vi "Testing.vi"() -> ()   [LabVIEW 2019]
panel:
  in  "process parameters":T1={"static gain"=2.5, "lag (s)"=2.5, "deadtime (s)"=0.001, "load"=0.0, "deadband"=0.0, "sensor noise"=0.0, "initial PV"=30.0, "plant noise"=0.0} {"plant noise" format="%.2f"; "initial PV" format="%.2f"; "sensor noise" format="%.2f"; "lag (s)" format="%.2f"; "deadtime (s)" format="%.2f"; "deadband" format="%.1f"; "load" format="%.2f"; "static gain" format="%.2f"}
  in  "PIDF gains":cluster{"Kp":dbl, "Ki":dbl, "Kd":dbl, "Kf":dbl}={"Kp"=5.0, "Ki"=0.0, "Kd"=0.0, "Kf"=0.0} {"Kf" format="%.3f"; "Kd" format="%.3f"; "Ki" format="%.3f"; "Kp" format="%.3f"}
  in  "output saturation range":cluster{"output high":dbl, "output low":dbl}={"output high"=inf, "output low"=-inf}
  in  "setpoint":dbl(slide) scale=-100.0..100.0
  out "Waveform Chart":T2(graph)
  in  "stop":bool
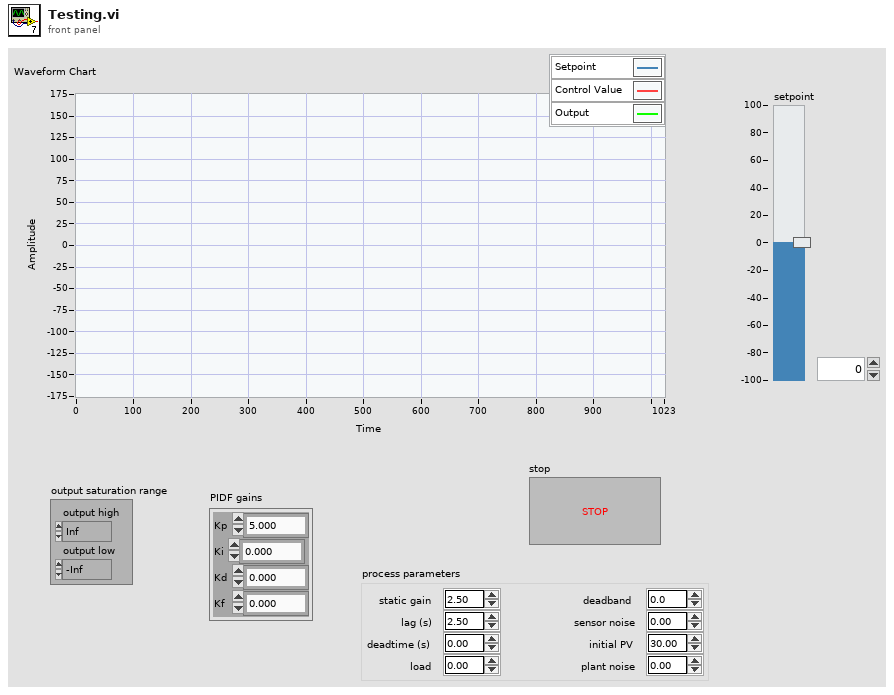
[diagram p1: front panel]
types:
  T1 = cluster{"static gain":dbl, "lag (s)":dbl, "deadtime (s)":dbl, "load":dbl, "deadband":dbl, "sensor noise":dbl, "initial PV":dbl, "plant noise":dbl}
  T2 = cluster{"setpoint":dbl, "output":dbl, "Plant Output":dbl}
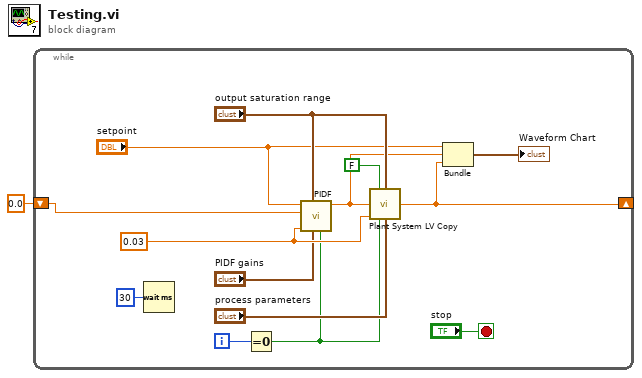
[diagram p0: block diagram]
diagram:
  n1 = while {
    shift-right: [w8] -> _
    shift-left: 0.0 ("Plant Output") -> [w10]
    i -> [w11]
    stop <- "stop" stop-if-true
    w13 = 0.03 ("dt (s)")
    n2 = Wait (ms)(milliseconds to wait=u32 30) -> ()  [unwired: 1 out]
    n3 = Equal To 0?(x=w11) -> (x = 0?=w3:bool)
    n4 = call "PIDF.vi"("reinitialize? (F)"=w3, "PIDF gains"="PIDF gains", "output range"="output saturation range", "dt (s)"=w13, "process variable"=w10, "setpoint"="setpoint") -> ("output"=w9:dbl)  [unwired: 3 in, 2 out]
    n5 = call "Plant System LV Copy.vi"("Integrator ?"=FALSE, "output saturation range"="output saturation range", "Plant Input"=w9, "dt (s)"=w13, "reinitialize? (F)"=w3, "process parameters"="process parameters") -> ("Plant Output"=w8:dbl)  [unwired: 9 in]
    n6 = Bundle("setpoint"="setpoint", "output"=w9, "Plant Output"=w8) -> (→"Waveform Chart":T2)  [unwired: 1 in]
  }
